vi "Target Lookup UFF Input.vi"(6 "Phase":dbl, 8 "Error In":errorcluster, 10 "Learning Gains":T1={"KL"=15.0, "Beta"=0.97, "D"=18}) -> (0 "UFF":dbl, 3 "Feed Forward for Display":dbl[](array[numeric]))   [LabVIEW 2018, in "COBRA Iterative Learning Control Library.lvlib"]
uses:
  COBRA Iterative Learning Control Library.lvlib
  Target Learning Gains.ctl
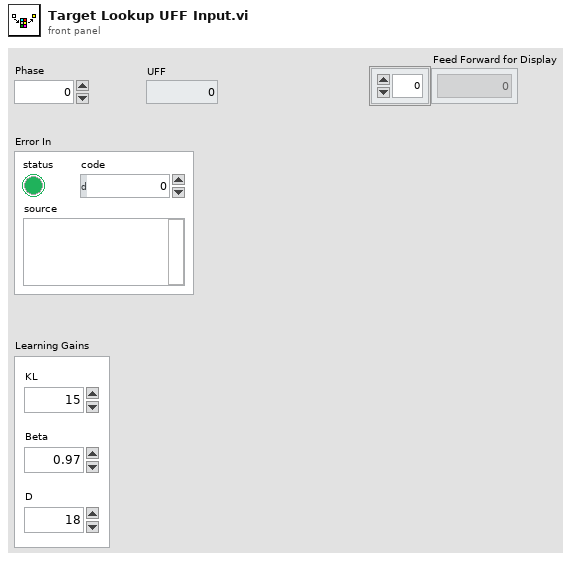
[diagram p1: front panel]
types:
  T1 = typedef "COBRA Iterative Learning Control Library.lvlib/Target Learning Gains.ctl" = cluster{"KL":dbl, "Beta":dbl, "D":i32}
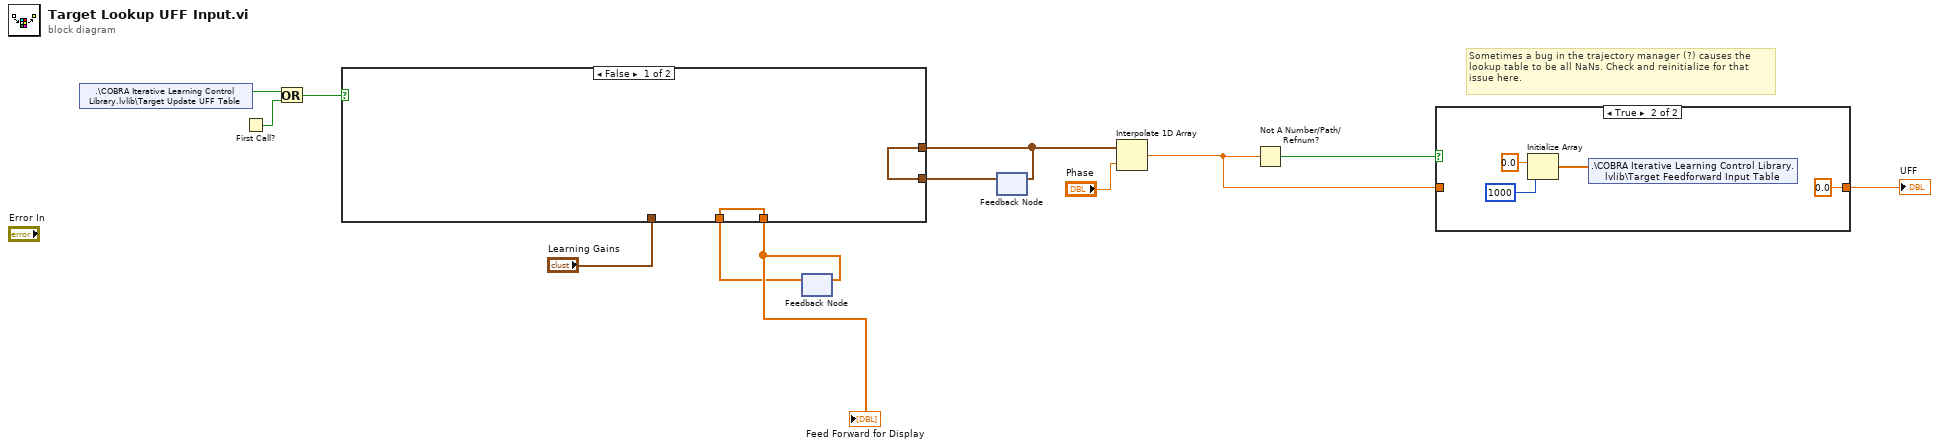
[diagram p0: block diagram]
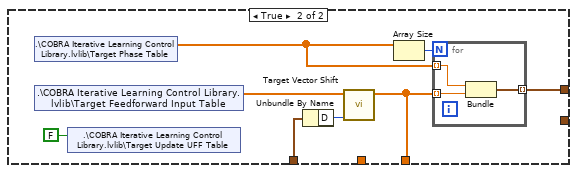
[diagram p3: hidden frame]
diagram:
  # "Sometimes a bug in the trajectory manager (?) causes the \nlookup table to be all NaNs. Check and reinitialize for that\nissue here."
  n1 = shared-variable ".\\COBRA Iterative Learning Control Library.lvlib\\Target Update UFF Table"() -> (w10:bool)  [unwired: 1 in, 1 out]
  n2 = First Call?() -> (First Call?: T/F=w11:bool)
  n3 = Or(x=w10, y=w11) -> (x .or. y?=w9:bool)
  n4 = feedback #1() -> (w1:dbl[])  [unwired: 1 in]
  n5 = feedback #2() -> (w8:cluster{"Numeric":dbl, "Numeric":dbl}[])  [unwired: 1 in]
  n6 = case shown="False" w9 {
    tunnel: [w14 w19] -> w7
    tunnel: w8 -> [w14 _]
    tunnel: "Learning Gains" -> [_ w17]
    tunnel: [w13 w15] -> w2
    tunnel: w1 -> [w13 _]
    frame False {
    }
    frame True {
      n7 = shared-variable ".\\COBRA Iterative Learning Control Library.lvlib\\Target Phase Table"() -> (w21:dbl[])  [unwired: 1 in, 1 out]
      n8 = shared-variable ".\\COBRA Iterative Learning Control Library.lvlib\\Target Feedforward Input Table"() -> (w18:dbl[])  [unwired: 1 in, 1 out]
      n9 = shared-variable ".\\COBRA Iterative Learning Control Library.lvlib\\Target Update UFF Table"(FALSE ("Update Lookup Tables")) -> ()  [unwired: 1 in, 1 out]
      n10 = Unbundle By Name(w17) -> ("D"=w16:i32)
      n11 = call "Target Vector Shift.vi"("Shift"=w16, "Input Vector"=w18) -> ("Output Vector"=w15:dbl[])  [unwired: 9 in]
      n12 = Array Size(array=w21) -> (size(s)=w22:i32)
      n13 = for {
        N: w22 -> [_]
        tunnel: w21 -> [w25] mode=indexing
        tunnel: w15 -> [w24] mode=indexing
        tunnel: [w23] -> w19 mode=indexing
        n14 = Bundle("Numeric"=w25, "Numeric"=w24) -> (w23:cluster{"Numeric":dbl, "Numeric":dbl})  [unwired: 1 in]
      }
    }
  }
  "Feed Forward for Display" <- w2
  n15 = feedback-in #1(w2) -> ()
  n16 = feedback-in #2(w7) -> ()
  n17 = Interpolate 1D Array(1:"Phase", 2:w7) -> (0:w4:dbl)
  n18 = Not A Number/Path/Refnum?(number/path/refnum=w4) -> (NaN/Path/Refnum?=w6:bool)
  n19 = case shown="True" w6 {
    tunnel: [w26 0.0 ("f")] -> w5
    tunnel: w4 -> [w26 _]
    frame False {
    }
    frame True {
      n20 = Initialize Array(0.0 ("element"), 1000 ("dimension size")) -> (w27:dbl[])
      n21 = shared-variable ".\\COBRA Iterative Learning Control Library.lvlib\\Target Feedforward Input Table"(w27) -> ()  [unwired: 1 in, 1 out]
    }
  }
  "UFF" <- w5
